vi "Sort Complex Numbers (obs).vi"(9 "method":u16(ring) items=["Real & Imaginary", "Magnitude"], 10 "order":enum16{"Ascending", "Descending"}(ring), 11 "Complex Numbers":cdb[](array[numeric]) format="%#.6g") -> (0 "error":i32, 2 "Sorted Index":i32[](array[numeric]), 3 "Sorted Complex Numbers":cdb[](array[numeric]) format="%#.6g")   [LabVIEW 2017, in "NI_AALPro.lvlib"]
uses:
  <vilib>/Analysis/NI_AALPro.lvlib
panel:
  # "This VI is obsolete !!!\nYou should replace this VI in your diagram with the Sort Complex Numbers VI.\n\nNOTE: If you set method to magnitude, please be aware that the new Sort \n            Complex Numbers VI sorts elements of the same magnitude first \n            with respect to their real parts and then with respect to their imaginary \n            parts."
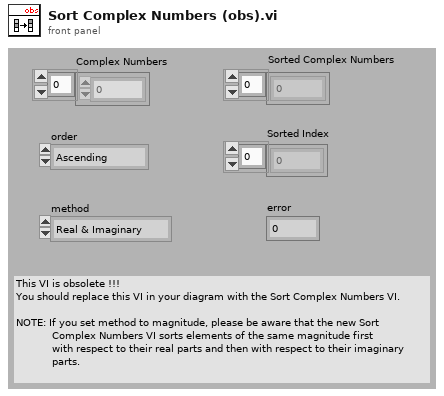
[diagram p1: front panel]
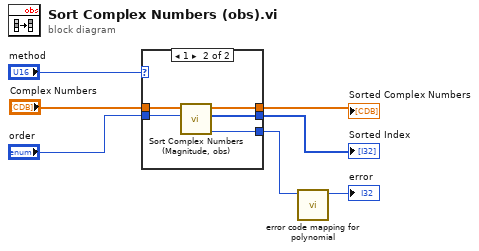
[diagram p0: block diagram]
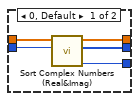
[diagram p2: hidden frame]
diagram:
  n1 = case shown="1" "method" {
    tunnel: "Complex Numbers" -> [w12 w17]
    tunnel: "order" -> [w11 w16]
    tunnel: [w10 w15] -> w4
    tunnel: [w9 w14] -> w3
    tunnel: [w8 w13] -> w2
    frame 0, Default {
      n2 = call <vilib>:"Sort Complex Numbers (Real&Imag).vi"("Order"=w11, "Complex Numbers"=w12) -> ("error"=w8:i32, "Sorted Index"=w9:i32[], "Sorted Complex Numbers"=w10:cdb[])  [unwired: 7 in]
    }
    frame 1 {
      n3 = call <vilib>:"Sort Complex Numbers (Magnitude, obs).vi"("Order"=w16, "Complex Numbers"=w17) -> ("error"=w13:i32, "Sorted Index"=w14:i32[], "Sorted Complex Numbers"=w15:cdb[])  [unwired: 7 in]
    }
  }
  "Sorted Complex Numbers" <- w4
  "Sorted Index" <- w3
  n4 = call <vilib>:"error code mapping for polynomial.vi"("error in"=w2) -> ("error out"=→"error":i32)  [unwired: 10 in]
